vi "ParamsProximiter.vi"(2 "paramsIn":variant) -> (16 "paramsOut":variant)   [LabVIEW 2017]
uses:
  Typedefs/Tipo_ParamsProximeter.ctl
  Typedefs/Tipo_ComponentesProximeter.ctl
panel:
  in  "Fase(º):":dbl
  in  "Distância Eixo:":dbl
  in  "120Hz":dbl caption="120 Hz:"
  in  "60Hz":dbl caption="60 Hz:"
  in  "0,45xRPM":dbl caption="0,45 x RPM:"
  in  "1/4xRPM":dbl caption="1/4 x RPM:"
  in  "1/3xRPM":dbl caption="1/3 x RPM:"
  in  "1/2xRPM":dbl caption="1/2 x RPM:"
  in  "3xRPM":dbl caption="3 x RPM:"
  in  "4xRPM":dbl caption="4 x RPM:"
  in  "2xRPM":dbl caption="2 x RPM:"
  in  "1xRPM":dbl caption="1 x RPM:"
  in  "Ruído:":dbl
  in  "Rotação (RPM):":dbl caption="RPM"
  in  "Init":bool
  # "Componentes:"
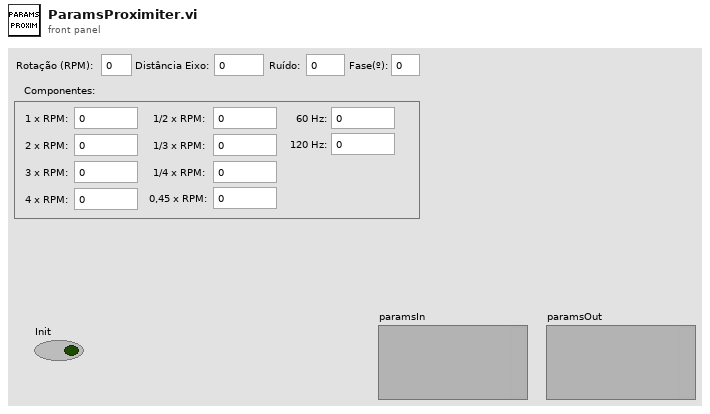
[diagram p1: front panel]
types:
  T1 = typedef "Tipo_ParamsProximeter.ctl" = cluster{"Rotacao":dbl, "Ruído":dbl, "Distância Eixo":dbl, "Fase":dbl, "Componentes":T2}
  T2 = typedef "Tipo_ComponentesProximeter.ctl" = cluster{"1xRPM":dbl, "2xRPM":dbl, "3xRPM":dbl, "4xRPM":dbl, "1/2xRPM":dbl, "1/3xRPM":dbl, "1/4xRPM":dbl, "0,45xRPM":dbl, "60Hz":dbl, "120Hz":dbl}
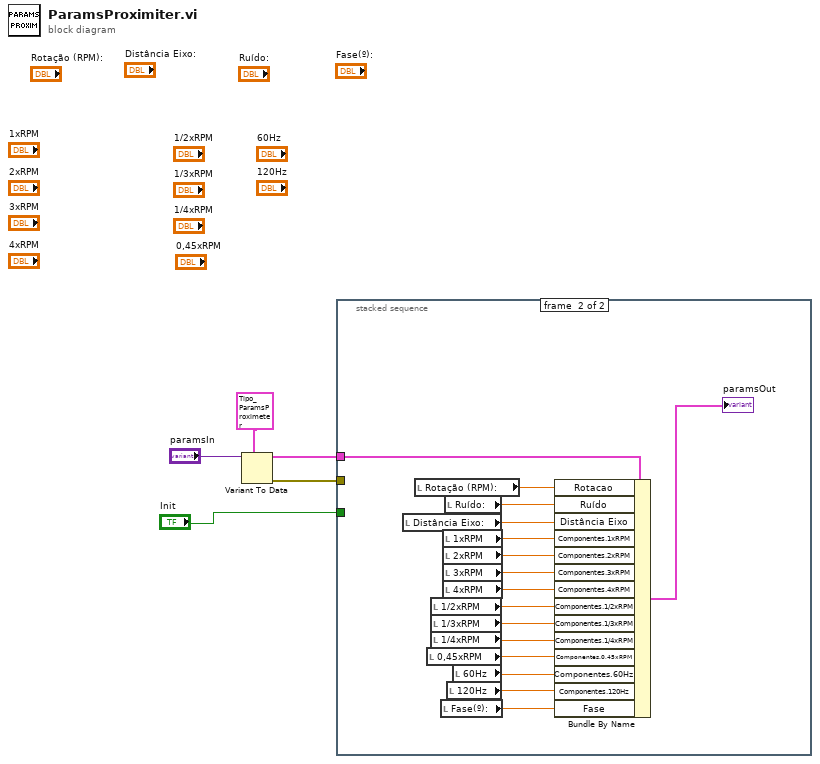
[diagram p0: block diagram]
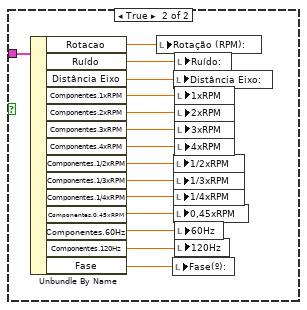
[diagram p3: hidden frame]
diagram:
  n1 = Variant To Data(type=T1 {"Rotacao"=0.0, "Ruído"=0.0, "Distância Eixo"=0.0, "Fase"=0.0, "Componentes"={"1xRPM"=0.0, "2xRPM"=0.0, "3xRPM"=0.0, "4xRPM"=0.0, "1/2xRPM"=0.0, "1/3xRPM"=0.0, "1/4xRPM"=0.0, "0,45xRPM"=0.0, "60Hz"=0.0, "120Hz"=0.0}} ("Tipo_ParamsProximeter"), Variant="paramsIn") -> (data=w4:T1, error out=w2:errorcluster)  [unwired: 1 in]
  n2 = stacked-sequence {
    tunnel: w4 -> [w7 w38]
    tunnel: "Init" -> [w6 _]
    tunnel: w2 -> [_ _]
    frame #0 {
      n3 = case shown="False" w6 {
        tunnel: w7 -> [_ w22]
        frame False {
        }
        frame True {
          n4 = Unbundle By Name(w22) -> ("Rotacao"=w21:dbl, "Ruído"=w20:dbl, "Distância Eixo"=w19:dbl, "Componentes.1xRPM"=w18:dbl, "Componentes.2xRPM"=w17:dbl, "Componentes.3xRPM"=w16:dbl, "Componentes.4xRPM"=w15:dbl, "Componentes.1/2xRPM"=w14:dbl, "Componentes.1/3xRPM"=w13:dbl, "Componentes.1/4xRPM"=w12:dbl, "Componentes.0,45xRPM"=w11:dbl, "Componentes.60Hz"=w10:dbl, "Componentes.120Hz"=w9:dbl, "Fase"=w8:dbl)
          n5 = local write "Rotação (RPM):"(w21) -> ()
          n6 = local write "Fase(º):"(w8) -> ()
          n7 = local write "Distância Eixo:"(w19) -> ()
          n8 = local write "1/2xRPM"(w14) -> ()
          n9 = local write "1/3xRPM"(w13) -> ()
          n10 = local write "1/4xRPM"(w12) -> ()
          n11 = local write "0,45xRPM"(w11) -> ()
          n12 = local write "Ruído:"(w20) -> ()
          n13 = local write "1xRPM"(w18) -> ()
          n14 = local write "2xRPM"(w17) -> ()
          n15 = local write "3xRPM"(w16) -> ()
          n16 = local write "4xRPM"(w15) -> ()
          n17 = local write "60Hz"(w10) -> ()
          n18 = local write "120Hz"(w9) -> ()
        }
      }
    }
    frame #1 {
      n19 = local read "Distância Eixo:"() -> (w35:dbl)
      n20 = local read "Rotação (RPM):"() -> (w37:dbl)
      n21 = local read "0,45xRPM"() -> (w27:dbl)
      n22 = local read "1/2xRPM"() -> (w30:dbl)
      n23 = local read "1/3xRPM"() -> (w29:dbl)
      n24 = local read "1/4xRPM"() -> (w28:dbl)
      n25 = local read "Fase(º):"() -> (w23:dbl)
      n26 = local read "1xRPM"() -> (w34:dbl)
      n27 = local read "2xRPM"() -> (w33:dbl)
      n28 = local read "3xRPM"() -> (w32:dbl)
      n29 = local read "4xRPM"() -> (w31:dbl)
      n30 = local read "Ruído:"() -> (w36:dbl)
      n31 = local read "120Hz"() -> (w25:dbl)
      n32 = local read "60Hz"() -> (w26:dbl)
      n33 = Bundle By Name(cluster=w38, "Rotacao"=w37, "Ruído"=w36, "Distância Eixo"=w35, "Componentes.1xRPM"=w34, "Componentes.2xRPM"=w33, "Componentes.3xRPM"=w32, "Componentes.4xRPM"=w31, "Componentes.1/2xRPM"=w30, "Componentes.1/3xRPM"=w29, "Componentes.1/4xRPM"=w28, "Componentes.0,45xRPM"=w27, "Componentes.60Hz"=w26, "Componentes.120Hz"=w25, "Fase"=w23) -> (→"paramsOut":T1)
    }
  }
